vi "bats.parser.runFpgaTests.vi"() -> (3 "All Passed?":bool)   [LabVIEW 2022 SP3]
panel:
  out "All compress.buffer":bool
  out "All test.parse.fields":bool
  out "All test.add.data.to.buffer":bool
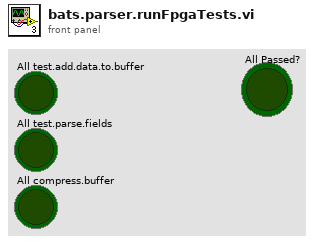
[diagram p1: front panel]
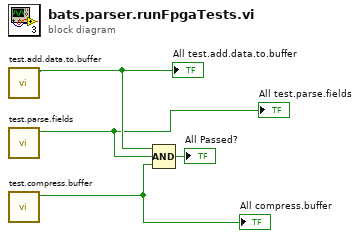
[diagram p0: block diagram]
diagram:
  n1 = call "test.add.data.to.buffer.vi"() -> ("All Passed"=w4:bool)  [unwired: 11 in]
  "All test.add.data.to.buffer" <- w4
  n2 = call "test.parse.fields.vi"() -> ("All Passed"=w3:bool)  [unwired: 11 in]
  "All test.parse.fields" <- w3
  n3 = call "test.compress.buffer.vi"() -> ("All Passed"=w1:bool)  [unwired: 11 in]
  "All compress.buffer" <- w1
  n4 = Compound Arithmetic op=AND(w4, w3, w1) -> (→"All Passed?":bool)
